vi "0_HomeAllAxes (SubVI).vi"(8 "error in (no error)":errorcluster) -> (0 "error out":errorcluster, 2 "Homed coordinates":T1, 3 "controller out":refnum<k24>, 5 "completed":bool)   [LabVIEW 2016]
doc: "Send all Aerotech axes (X, Y, Z) to their home positions [ (0,0,0) mm ] at the specified homing speed [ (25,10, 10) mm/s ]. \n\nSteps: \n\n1. Connect to the Aerotech XYZ stage\n2. Enable all axes. While enabled, the axes are locked in place, and vary by <0.2 um from their positions. Disabling the axes unlocks them, allowing them to vary by as much as 0.5 um from their given positions. As such, axes must be enabled for the full length of stage construction.\n3. Move to the home position (here, designated as 0, 0, 0). \"Wait\" prevents us from taking another action until the machine completes the move.\n4. Mark the Home position. This Aerotech vi, \"Home,\" initiates the autocalibration sequence for the stage. \n5. Wait - Home - Get Position: cross check the homing sequence result\n6. Output the controller refnum and any errors. A boolean indicator will also show that the homing sequence is complete, and we can print the current coordinates. \n\nBuilt on top of the Aerotech .NET libraries."
uses:
  C:/Users/sciollalab/Documents/Brandeis-BNL/LabVIEW_Codes/BNLStaveAssembly-Blueprint/Bin/Aerotech.A3200.dll
  BNLStaveAssembly-Blueprint/Bin/Aerotech.A3200.dll
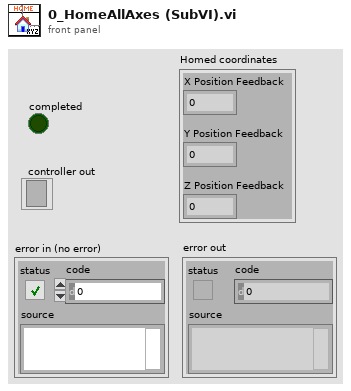
[diagram p1: front panel]
types:
  T1 = cluster{"X Position Feedback":dbl, "Y Position Feedback":dbl, "Z Position Feedback":dbl}
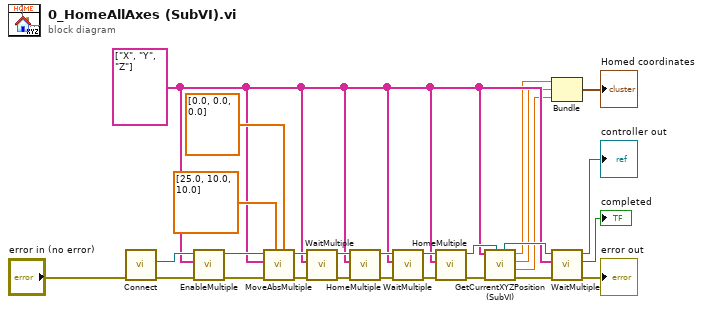
[diagram p0: block diagram]
diagram:
  w6 = string[] ["X", "Y", "Z"] ("axis names")
  n1 = call "Connect.vi"("error in (no error)"="error in (no error)") -> ("error out"=w25:errorcluster, "controller"=w26:refnum<k24>)  [unwired: 9 in]
  n2 = call "EnableMultiple.vi"("error in (no error)"=w25, "axis names"=w6, "controller in"=w26) -> ("error out"=w21:errorcluster, "controller out"=w22:refnum<k24>)  [unwired: 7 in]
  n3 = call "MoveAbsMultiple.vi"("positions"=dbl[] [0.0, 0.0, 0.0], "speeds"=dbl[] [25.0, 10.0, 10.0], "error in (no error)"=w21, "axis names"=w6, "controller in"=w22) -> ("error out"=w20:errorcluster, "controller out"=w19:refnum<k24>)  [unwired: 5 in]
  n4 = call "WaitMultiple.vi"("error in (no error)"=w20, "axis names"=w6, "controller in"=w19) -> ("error out"=w17:errorcluster, "controller out"=w18:refnum<k24>)  [unwired: 6 in, 1 out]
  n5 = call "HomeMultiple.vi"("error in (no error)"=w17, "axis names"=w6, "controller in"=w18) -> ("error out"=w15:errorcluster, "controller out"=w16:refnum<k24>)  [unwired: 7 in]
  n6 = call "WaitMultiple.vi"("error in (no error)"=w15, "axis names"=w6, "controller in"=w16) -> ("error out"=w13:errorcluster, "controller out"=w14:refnum<k24>)  [unwired: 6 in, 1 out]
  n7 = call "HomeMultiple.vi"("error in (no error)"=w13, "axis names"=w6, "controller in"=w14) -> ("error out"=w12:errorcluster, "controller out"=w11:refnum<k24>)  [unwired: 7 in]
  n8 = call "GetCurrentXYZPosition (SubVI).vi"(".NET Refnum in - Device"=w11, "error in (no error)"=w12, "Axes Names"=w6) -> ("error out"=w7:errorcluster, "Z Position Feedback"=w3:dbl, "Y Position Feedback"=w4:dbl, "X Position Feedback"=w5:dbl, ".NET Refnum out  - Device"=w8:refnum<k24>)  [unwired: 3 in, 1 out]
  n9 = Bundle("X Position Feedback"=w5, "Y Position Feedback"=w4, "Z Position Feedback"=w3) -> (→"Homed coordinates":T1)  [unwired: 1 in]
  n10 = call "WaitMultiple.vi"("error in (no error)"=w7, "axis names"=w6, "controller in"=w8) -> ("error out"=→"error out":errorcluster, "completed"=→"completed":bool, "controller out"=→"controller out":refnum<k24>)  [unwired: 6 in]
